vi "DeCoF boolean query.vi"(4 "error in":errorcluster, 5 "use gsv":bool, 6 "param-name":string, 7 "Conncection ID in":T1) -> (0 "error out":errorcluster, 2 "value":bool, 3 "Conncection ID out":T1)   [LabVIEW 2013]
uses:
  subVIs/DeCoF connection.ctl
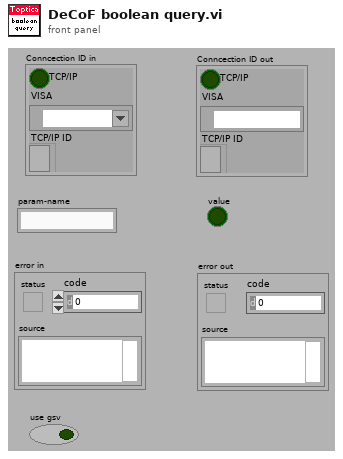
[diagram p1: front panel]
types:
  T1 = typedef "DeCoF connection.ctl" = cluster{"TCP/IP":bool, "VISA":refnum<visa-resource-name>, "TCP/IP ID":refnum<k5>}
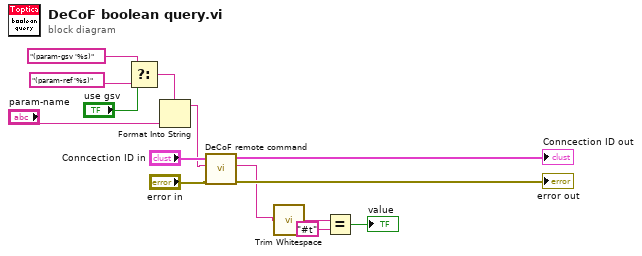
[diagram p0: block diagram]
diagram:
  n1 = Select(t="(param-gsv '%s)" ("format string"), s="use gsv", f="(param-ref '%s)" ("format string")) -> (s? t:f=w8:string)
  n2 = Format Into String(format string=w8, "param-name") -> (resulting string=w5:string)  [unwired: 2 in, 1 out]
  n3 = call "DeCoF remote command.vi"("error in (no error)"="error in", "command"=w5, "Conncection ID in"="Conncection ID in") -> ("error out"=→"error out":errorcluster, "answer string"=w4:string, "Conncection ID out"=→"Conncection ID out":T1)  [unwired: 2 in, 2 out]
  n4 = call <vilib>:"Trim Whitespace.vi"("string"=w4) -> ("trimmed string"=w3:string)  [unwired: 1 in]
  n5 = Equal?(x=w3, y="#t") -> (x = y?=→"value":bool)
